vi "Timed log record .vi"(9 "log input":string, 10 "system":string="S4ICS", 11 "type":T1(ring)) -> (2 "log register":string, 3 "timestamp":string)   [LabVIEW 2018]
panel:
  # "ISO 8601:\nSeptember 27, 2022 at 6 p.m. is represented as 2022-09-27T18:00:00.000"
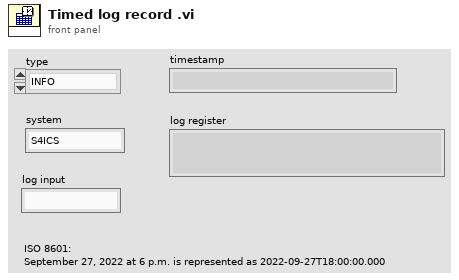
[diagram p1: front panel]
types:
  T1 = enum16{"INFO", "TRACE", "DEBUG", "WARN", "ERROR", "FATAL", "OTHER"}
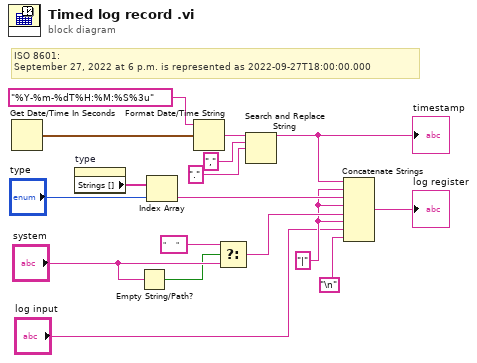
[diagram p0: block diagram]
diagram:
  w4 = "|"
  # "ISO 8601:\nSeptember 27, 2022 at 6 p.m. is represented as 2022-09-27T18:00:00.000"
  n1 = Get Date/Time In Seconds() -> (seconds since 1Jan1904=w13:timestamp)
  n2 = property on="type" class="Enum (strict)"() -> ("Strings []"=w9:string[])  [unwired: 2 in, 2 out]
  n3 = Empty String/Path?(string/path="system") -> (empty?=w10:bool)
  n4 = Index Array(array=w9, index="type") -> (element=w6:string)
  n5 = Format Date/Time String(time format string (%c)="%Y-%m-%dT%H:%M:%S%3u", seconds (now)=w13) -> (date/time string=w16:string)  [unwired: 1 in]
  n6 = Select(t="     ", s=w10, f="system") -> (s? t:f=w5:string)
  n7 = Search and Replace String(input string=w16, search string=",", replace string=".") -> (result string=w7:string)  [unwired: 5 in, 3 out]
  "timestamp" <- w7
  n8 = Concatenate Strings(w7, w4, w6, w4, w5, w4, "log input", "\n") -> (→"log register":string)
